vi "PRL STR Convert SGL Array to String.vi"(10 "Precision":i32, 11 "Values":sgl[](array[numeric])) -> (3 "Strings":string[](array[string]))   [LabVIEW 2013, in "PMU Recorder Light.lvlib"]
uses:
  PMU Recorder Light.lvlib
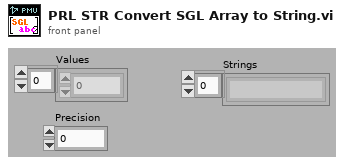
[diagram p1: front panel]
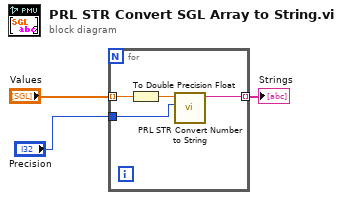
[diagram p0: block diagram]
diagram:
  n1 = for {
    tunnel: "Values" -> [w7] mode=indexing
    tunnel: "Precision" -> [w5]
    tunnel: [w4] -> w1 mode=indexing
    n2 = To Double Precision Float(number=w7) -> (double precision float=w6:dbl)
    n3 = call "PRL STR Convert Number to String.vi"("Precision"=w5, "Number"=w6) -> ("Number String"=w4:string)  [unwired: 9 in]
  }
  "Strings" <- w1
